vi "Delete Tags.vi"(8 "error in (no error)":errorcluster, 10 "Tag":string[](array[string]), 11 "File Tree In":refnum<class "File Tree.lvclass">) -> (0 "error out":errorcluster, 3 "File Tree Out":refnum<class "File Tree.lvclass">)   [LabVIEW 2020, in "Tree Helpers.lvlib" / "File Tree.lvclass"]
uses:
  File Tree.lvclass
  File Tree.lvclass/File Tree.ctl
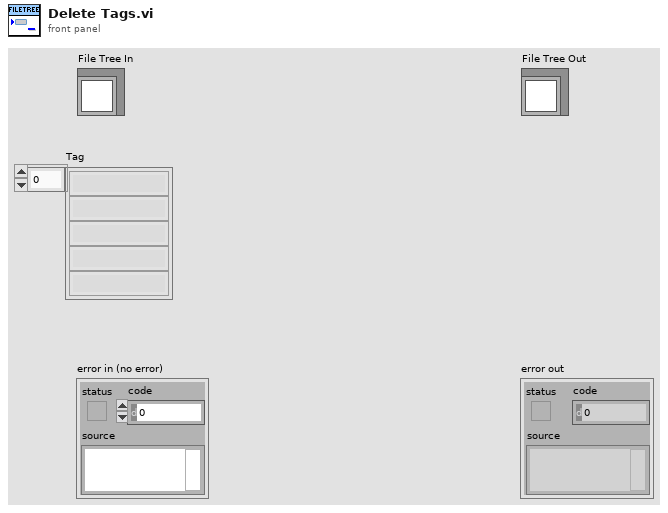
[diagram p1: front panel]
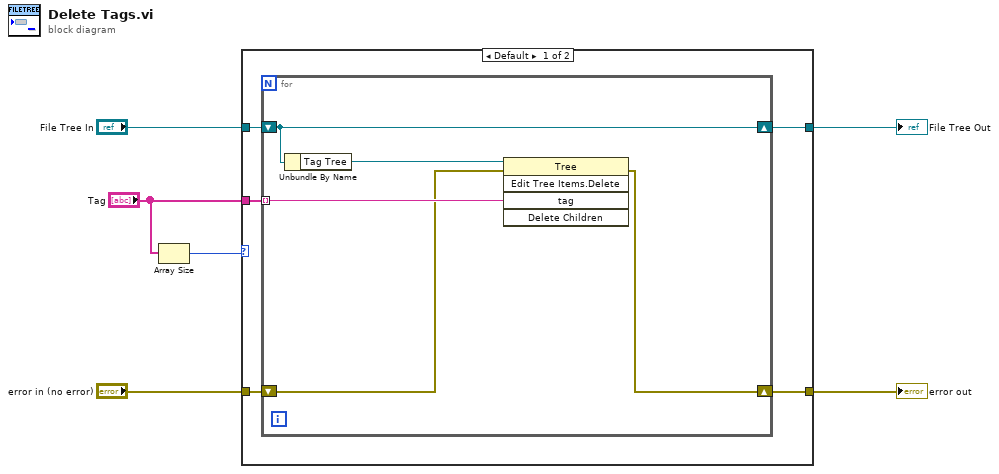
[diagram p0: block diagram]
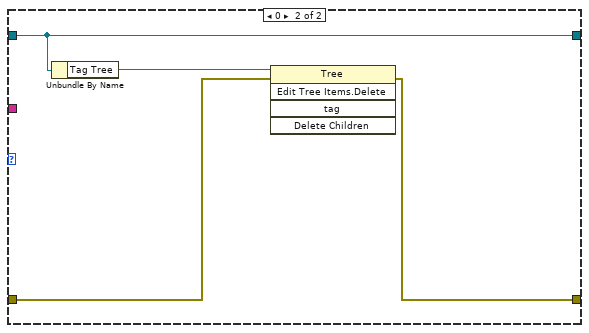
[diagram p2: hidden frame]
diagram:
  n1 = Array Size(array="Tag") -> (size(s)=w1:i32)
  n2 = case shown="Default" w1 {
    tunnel: "File Tree In" -> [w11 w20]
    tunnel: "error in (no error)" -> [w10 w19]
    tunnel: [w9 w18] -> w4
    tunnel: [w8 w20] -> w3
    tunnel: "Tag" -> [w7 _]
    frame Default {
      n3 = for {
        tunnel: w7 -> [w15] mode=indexing
        shift-right: [w13] -> w9
        shift-left: w10 -> [w14]
        shift-right: [w12] -> w8
        shift-left: w11 -> [w12]
        n4 = Unbundle By Name(w12) -> ("Tag Tree"=w16:refnum<vi>)
        n5 = invoke class="Tree" method="Edit Tree Items.Delete"(reference=w16, error in=w14, "tag"=w15) -> (error out=w13:errorcluster)  [unwired: 2 in, 4 out]
      }
    }
    frame 0 {
      n6 = Unbundle By Name(w20) -> ("Tag Tree"=w17:refnum<vi>)
      n7 = invoke class="Tree" method="Edit Tree Items.Delete"(reference=w17, error in=w19) -> (error out=w18:errorcluster)  [unwired: 3 in, 4 out]
    }
  }
  "error out" <- w4
  "File Tree Out" <- w3
